vi "SGDA-Get Device Properties.vi"(0 "Hardware Config In":T5={"TDT"={"Output"={"Device"=enum."None", "Num"=0}, "Input"=enum."Front Panel"}, "Transducer"="", "Properties"={"Amplifier"=enum."None", "Panic button"=FALSE}, "System"=enum."PXI"}, 7 "Eclipse":T1) -> (4 "Num Inputs":i32, 6 "Gain":dbl)   [LabVIEW 2020]
uses:
  EPhys/LV Source/Typedefs/EPhys-Hardware Config.ctl
  TDT VIs/Typedefs/TDT-Device Config.ctl
  TDT VIs/Typedefs/TDT-Output source.ctl
  TDT VIs/Typedefs/TDT-Device ID.ctl
  TDT VIs/Typedefs/TDT-Input source.ctl
  EPhys/LV Source/Typedefs/EPhys-Hardware Properties.ctl
  Type Defs/Hardware Destination.ctl
  EPhys/LV Source/Typedefs/EPhys-Eclipse Settings.ctl
  EPhys/LV Source/Typedefs/EPhys-Eclipse Lowpass.ctl
  EPhys/LV Source/Typedefs/EPhys-Eclipse Highpass.ctl
  EPhys/LV Source/Typedefs/EPhys-Eclipse Gain.ctl
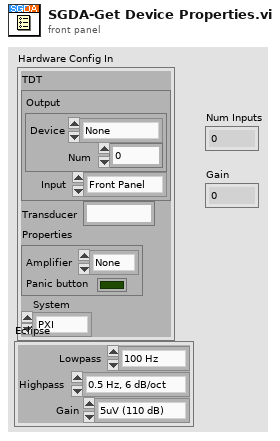
[diagram p1: front panel]
types:
  T1 = typedef "EPhys-Eclipse Settings.ctl" = cluster{"Lowpass":T2, "Highpass":T3, "Gain":T4}
  T2 = typedef "EPhys-Eclipse Lowpass.ctl" = enum16{"100 Hz", "300 Hz", "750 Hz", "1000 Hz", "1500 Hz", "2000 Hz", "3000 Hz", "4000 Hz", "5000 Hz", "7500 Hz"}
  T3 = typedef "EPhys-Eclipse Highpass.ctl" = enum16{"0.5 Hz, 6 dB/oct", "1 Hz, 6 dB/oct", "3.3 Hz, 6 dB/oct", "10 Hz, 6 dB/oct", "33 Hz, 6 dB/oct", "100 Hz, 6 dB/oct", "10 Hz, 12 dB/oct", "100 Hz, 12 dB/oct"}
  T4 = typedef "EPhys-Eclipse Gain.ctl" = enum16{"5uV (110 dB)", "6uV (108 dB)", "7uV (107 dB)", "8uV (106 dB)", "9uV (105 dB)", "10uV (104 dB)", "20uV (98 dB)", "40uV (92 dB)", "80uV (86 dB)", "160uV (80 dB)", "320uV (74 dB)"}
  T5 = typedef "EPhys-Hardware Config.ctl" = cluster{"TDT":T6, "Transducer":string, "Properties":T10, "System":T11}
  T6 = typedef "TDT-Device Config.ctl" = cluster{"Output":T7, "Input":T9}
  T7 = typedef "TDT-Output source.ctl" = cluster{"Device":T8, "Num":i32}
  T8 = typedef "TDT-Device ID.ctl" = enum16{"None", "PA5", "RP2", "RL2", "RA16", "RV8", "RX5", "RX6", "RX7", "RX8", "RZ2", "RZ5", "RZ6"}
  T9 = typedef "TDT-Input source.ctl" = enum16{"Front Panel", "RA4LI", "RA16LI"}
  T10 = typedef "EPhys-Hardware Properties.ctl" = cluster{"Amplifier":enum16{"None", "Biosemi", "Eclipse", "Eclipse (N.C.)", "Grass"}, "Panic button":bool}
  T11 = typedef "Hardware Destination.ctl" = enum16{"None", "PXI", "TDT", "NI", "TDTSIM"}
  T12 = enum16{"None", "Biosemi", "Eclipse", "Eclipse (N.C.)", "Grass"}
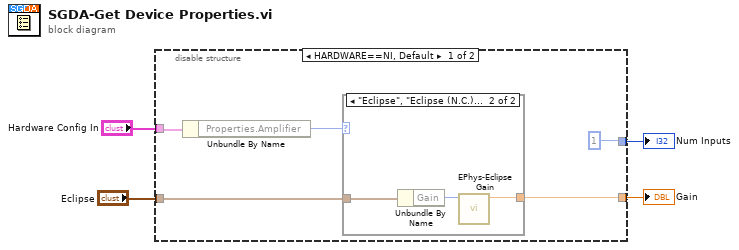
[diagram p0: block diagram]
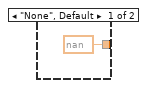
[diagram p2: hidden frame]
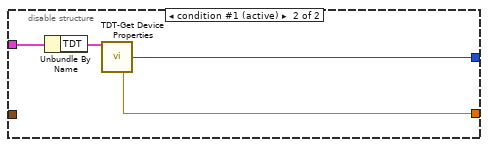
[diagram p3: hidden frame]
diagram:
  n1 = disable-structure shown="HARDWARE==NI, Default" {
    disable-tunnel: [w9 w17] -> w4
    disable-tunnel: [1 w16] -> w3
    disable-tunnel: "Hardware Config In" -> [w6 w14]
    disable-tunnel: "Eclipse" -> [w7 _]
    frame condition #0 {
      n2 = Unbundle By Name(w6) -> ("Properties.Amplifier"=w5:T12)
      n3 = case shown="\"Eclipse\", \"Eclipse (N.C.)\"" w5 {
        tunnel: [nan ("Gain out") w13] -> w9
        tunnel: w7 -> [_ w12]
        frame "None", Default {
        }
        frame "Eclipse", "Eclipse (N.C.)" {
          n4 = Unbundle By Name(w12) -> ("Gain"=w11:T4)
          n5 = call "EPhys-Eclipse Gain.vi"("Gain in"=w11) -> ("Gain out"=w13:dbl)  [unwired: 9 in, 1 out]
        }
      }
    }
    frame condition #1 (active) {
      n6 = Unbundle By Name(w14) -> ("TDT"=w15:T6)
      n7 = call "TDT-Get Device Properties.vi"("TDT-Device Config"=w15) -> ("Num Inputs"=w16:i32, "Gain"=w17:dbl)  [unwired: 9 in, 4 out]
    }
  }
  "Gain" <- w4
  "Num Inputs" <- w3
